vi "Packetize b.vi"(0 "Arduino Resource in":T3, 7 "Data":u8[](array[numeric]), 11 "error in":errorcluster) -> (4 "Arduino Resource out":T3, 8 "Packet":string, 15 "error out":errorcluster)   [LabVIEW 2015]
doc: "Pack data into packets including checksum and ensure fixed packet length."
uses:
  <vilib>/LabVIEW Interface for Arduino/Type Defs/Board Type.ctl
  <vilib>/LabVIEW Interface for Arduino/Type Defs/Connection Type.ctl
  <vilib>/LabVIEW Interface for Arduino/LabVIEW Interface for Arduino.lvlib
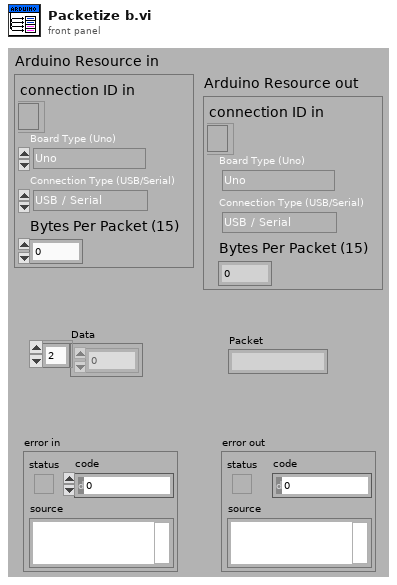
[diagram p1: front panel]
types:
  T1 = typedef "LabVIEW Interface for Arduino.lvlib/Board Type.ctl" = enum16{"Uno", "Dimuelanove w/Atmega 328", "Mega 2560"}
  T2 = typedef "LabVIEW Interface for Arduino.lvlib/Connection Type.ctl" = enum8{"USB / Serial", "XBEE", "BlueSmirf (Bluetooth)"}
  T3 = cluster{"connection ID in":refnum<k31>, "Board Type (Uno)":T1, "Connection Type (USB/Serial)":T2, "Bytes Per Packet (15)":u32}
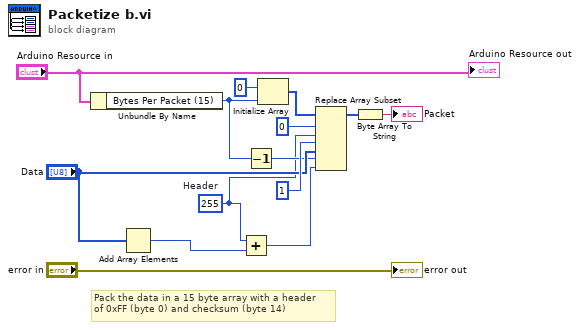
[diagram p0: block diagram]
diagram:
  w2 = u8 255  # Header
  # "Pack the data in a 15 byte array with a header \nof 0xFF (byte 0) and checksum (byte 14)"
  n1 = Unbundle By Name("Arduino Resource in") -> ("Bytes Per Packet (15)"=w5:u32)
  n2 = Add Array Elements(numeric array="Data") -> (sum=w3:u8)
  n3 = Add(x=w2, y=w3) -> (x+y=w8:u8)
  n4 = Decrement(x=w5) -> (x-1=w6:u32)
  n5 = Initialize Array(u8 0, w5) -> (w14:u8[])
  n6 = Replace Array Subset(array=w14, new element #1=w2, index #1=0 ("index"), new element #2="Data", index #2=1 ("index"), new element #3=w8, index #3=w6) -> (w7:u8[])
  n7 = Byte Array To String(unsigned byte array=w7) -> (string=→"Packet":string)
  "error out" <- "error in"
  "Arduino Resource out" <- "Arduino Resource in"
